vi "get map wall coordinate.vi"(8 "error in (no error)":errorcluster, 11 "data array":string[](array[string])) -> (0 "error out":errorcluster, 3 "Array":cluster{cluster{"X":dbl, "Y":dbl}[]}[](array[cluster]))   [LabVIEW 2019]
uses:
  <vilib>/JDP Science/JSONtext/Find Item.vi
  <vilib>/JDP Science/JSONtext/String Subset.vi
  <vilib>/JDP Science/JSONtext/Offset/Find Object Item Locations by Names.vi
  <vilib>/JDP Science/JSONtext/support/Quote and Escape JSON string.vi
  <vilib>/JDP Science/JSONtext/Parsing/Advance past whitespace.vi
  <vilib>/JDP Science/JSONtext/support/Commas Needed.vi
  <vilib>/JDP Science/JSONtext/Parsing/Advance past whitespace and comma.vi
  <vilib>/JDP Science/JSONtext/Parsing/Advance past next JSON Value (inlined COPY).vi
  <vilib>/JDP Science/JSONtext/Parsing/Advance past Item Name.vi
  <vilib>/JDP Science/JSONtext/support/quote and escape json string 2.vi
  <vilib>/JDP Science/JSONtext/Parsing/Advance past Line Ending.vi
  <vilib>/JDP Science/JSONtext/Parsing/Advance past String.vi
  <vilib>/JDP Science/JSONtext/Parsing/Advance past Number.vi
  <vilib>/JDP Science/JSONtext/Parsing/Parse Full Path or Item Name.vi
  <vilib>/JDP Science/JSONtext/Next JSON Value.vi
  <vilib>/JDP Science/JSONtext/support/Error Cluster From Code.vi
  <vilib>/JDP Science/JSONtext/Offset/Find Item Locations by Path.vi
  <vilib>/JDP Science/JSONtext/Parsing/Advance past Array.vi
  <vilib>/JDP Science/JSONtext/Parsing/Advance past Object.vi
  <vilib>/JDP Science/JSONtext/Parsing/Parsing Error.vi
  <vilib>/JDP Science/JSONtext/JSONtext.lvlib
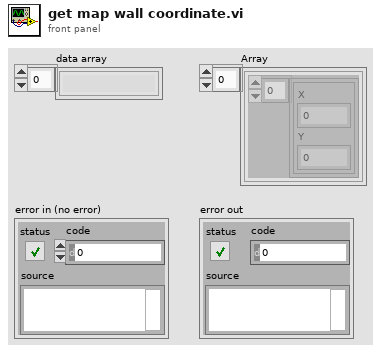
[diagram p1: front panel]
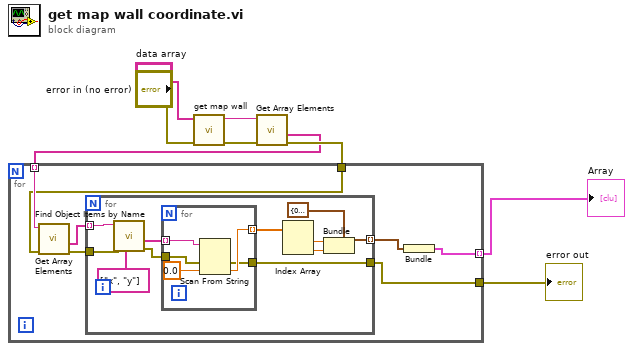
[diagram p0: block diagram]
diagram:
  n1 = call "get map wall.vi"("error in (no error)"="error in (no error)", "data array"="data array") -> ("error out"=w3:errorcluster, "<JSON> wall array"=w4:string)  [unwired: 8 in]
  n2 = call <vilib>:"Get Array Elements.vi"("error in (no error)"=w3, "JSON"=w4) -> ("error out"=w7:errorcluster, "<JSON>"=w5:string[])  [unwired: 7 in, 1 out]
  n3 = for {
    tunnel: w5 -> [w14] mode=indexing
    tunnel: [w12] -> w6 mode=indexing
    tunnel: w7 -> [w11]
    tunnel: [w9] -> w8
    n4 = call <vilib>:"Get Array Elements.vi"("error in (no error)"=w11, "JSON"=w14) -> ("error out"=w10:errorcluster, "<JSON>"=w15:string[])  [unwired: 7 in, 1 out]
    n5 = for {
      tunnel: w15 -> [w26] mode=indexing
      tunnel: [w22] -> w13 mode=indexing
      tunnel: w10 -> [w18]
      tunnel: [w16] -> w9
      n6 = call <vilib>:"Find Object Items by Name.vi"("Item Names"=string[] ["x", "y"], "error in (no error)"=w18, "JSON"=w26) -> ("error out"=w17:errorcluster, "<JSON>"=w21:string[])  [unwired: 6 in, 1 out]
      n7 = for {
        tunnel: w21 -> [w31] mode=indexing
        tunnel: [w30] -> w20 mode=indexing
        tunnel: w17 -> [w28]
        tunnel: [w27] -> w16
        n8 = Scan From String(input string=w31, error in=w28, default 1=0.0) -> (error out=w27:errorcluster, output 1=w30:dbl)  [unwired: 2 in, 2 out]
      }
      n9 = Index Array(array=w20) -> (element #1=w23:dbl, element #2=w24:dbl)  [unwired: 2 in]
      n10 = Bundle(cluster=cluster{"X":dbl, "Y":dbl} {"X"=0.0, "Y"=0.0} ("Cluster"), "X"=w23, "Y"=w24) -> (w22:cluster{"X":dbl, "Y":dbl})
    }
    n11 = Bundle(w13) -> (w12:cluster{cluster{"X":dbl, "Y":dbl}[]})  [unwired: 1 in]
  }
  "error out" <- w8
  "Array" <- w6
